vi "Example_Labview.vi"() -> ()   [LabVIEW 2019]
uses:
  <vilib>/myRIO/Common/Instrument Driver Framework/Utilities/typedefs/Analog Scaling Constants.ctl
  <vilib>/myRIO/Common/Instrument Driver Framework/Utilities/typedefs/Analog Scaling Constants List.ctl
  <vilib>/myRIO/Common/Instrument Driver Framework/myRIO v1.0/AO/typedefs/AO Channels Enum.ctl
  <vilib>/myRIO/Common/Instrument Driver Framework/myRIO v1.0/AO/typedefs/AO Channels List.ctl
  <vilib>/myRIO/Common/Instrument Driver Framework/Utilities/typedefs/Generic FPGA Reference.ctl
  <vilib>/myRIO/Common/Instrument Driver Framework/Utilities/typedefs/myRIO v1.0 Reference.ctl
  <vilib>/myRIO/Common/Instrument Driver Framework/Utilities/typedefs/Hardware Version Enum.ctl
  <vilib>/myRIO/Common/Instrument Driver Framework/Utilities/typedefs/myRIO Generic Hardware Reference.ctl
  <vilib>/myRIO/Instrument Drivers/Onboard IO/AO/typedefs/AO Reference.ctl
  <vilib>/userdefined/High Color/nirio_resource_hc.ctl
  <vilib>/myRIO/Common/Instrument Driver Framework/myRIO v1.0/AO/vis/myRIO v1.1 Open AO.vi
  <vilib>/myRIO/Instrument Drivers/Onboard IO/AO/vis/myRIO AO Open.xnode
  <vilib>/myRIO/Common/Instrument Driver Framework/myRIO v1.0/Encoder/typedefs/Encoder Signal Mode.ctl
  <vilib>/myRIO/Common/Instrument Driver Framework/myRIO v1.0/AI/typedefs/AI Channels Enum.ctl
  <vilib>/myRIO/Common/Instrument Driver Framework/myRIO v1.0/AI/typedefs/AI Channels List.ctl
  <vilib>/myRIO/Instrument Drivers/Onboard IO/AI/typedefs/AI Reference.ctl
  <vilib>/myRIO/Common/Instrument Driver Framework/myRIO v1.0/AI/vis/myRIO v1.1 Open AI.vi
  <vilib>/myRIO/Instrument Drivers/Onboard IO/AI/vis/myRIO AI Open.xnode
  <vilib>/Platform/TimedLoop/XDataNode/XDataNode.xnode
  <vilib>/Platform/TimedLoop/XDataNode/nitl_modes.ctl
  <vilib>/Platform/TimedLoop/XDataNode/XDNodeRunTimeDep.lvlib
  <vilib>/Platform/TimedLoop/XDataNode/wakeup.ctl
  <vilib>/Platform/TimedLoop/XDataNode/timing_clust.ctl
  <vilib>/Analysis/3filter.llb/Filter Passband Type.ctl
  <vilib>/Analysis/NI_AALBase.lvlib
  <vilib>/ptbypt/NI_PtbyPt.lvlib
  Shared VIs/TypeDef_TDMS_States.ctl
panel:
  out "Current [A]":dbl
  out "Voltage":dbl
  out "Time (ms)":dbl
  out "Velocity encoder LP [deg/s]":dbl
  out "Velocity unfiltered [deg/s]":dbl
  out "Force unfiltered [N]":dbl
  in  "File name":string
  in  "Stop saving data":bool
  in  "Save data?":bool
  out "Force [N]":dbl
  out "Force Chart":dbl(graph)
  out "Velocity [deg/s]":dbl
  out "Velocity Chart":dbl(graph)
  out "Position [deg]":dbl
  out "Position Chart":dbl(graph)
  in  "stop":bool
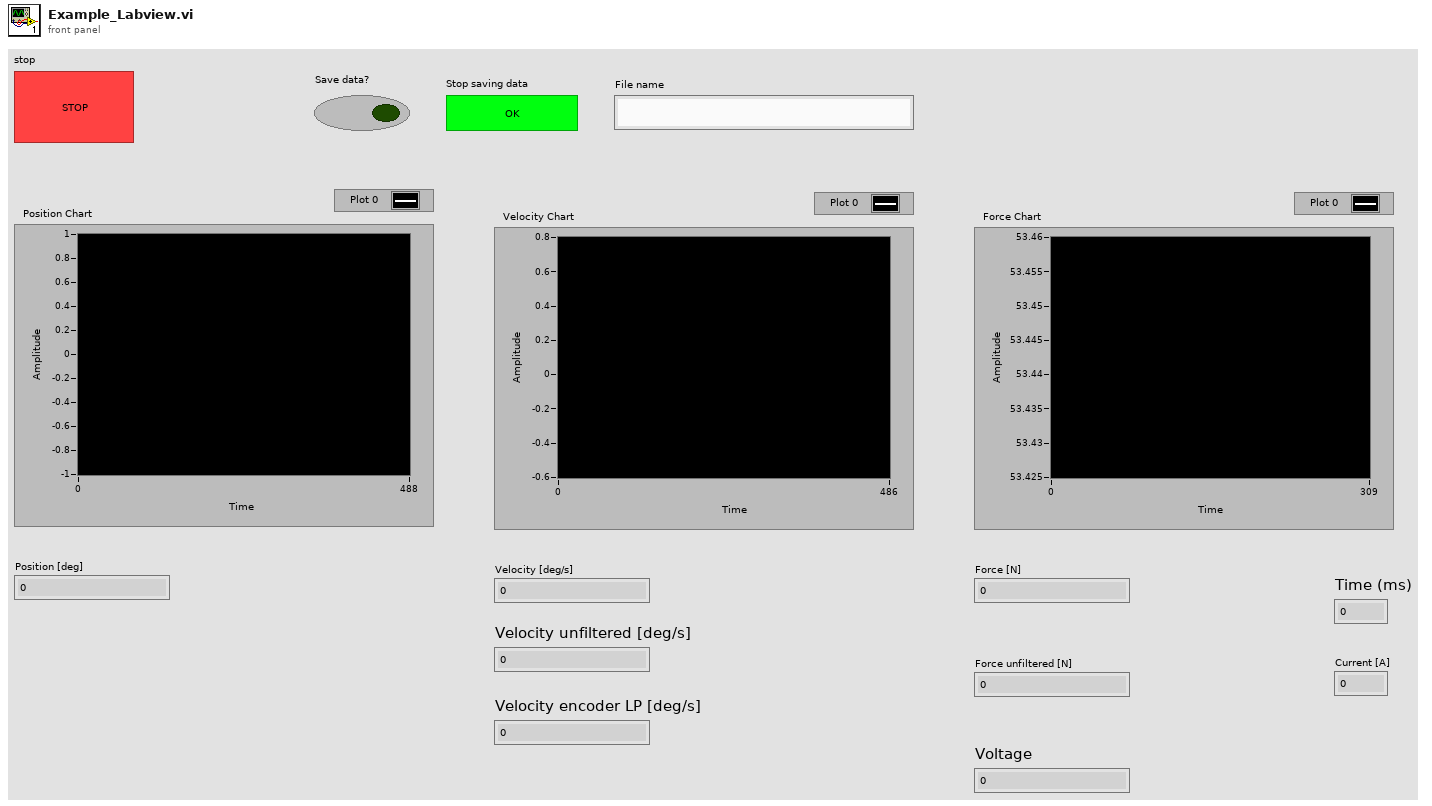
[diagram p1: front panel]
types:
  T1 = typedef "nirio_resource_hc.ctl" = tag
  T2 = typedef "Hardware Version Enum.ctl" = enum16{"Unknown", "myRIO-1900", "myRIO-1950", "roboRIO"}
  T3 = typedef "TypeDef_TDMS_States.ctl" = enum16{"Do Nothing", "Create", "Write", "Close"}
  T4 = enum16{"open", "open or create", "create or replace", "create", "open (read-only)"}
  T5 = typedef "XDNodeRunTimeDep.lvlib/timing_clust.ctl" = cluster{"Expected End [f-1]":u64, "Actual End [f-1]":u64, "Finished Late? [f-1]":bool, "Expected End [i-1]":u64, "Actual End [i-1]":u64, "Finished Late? [i-1]":bool, "Expected Start [i]":u64, "Actual Start [i]":u64, "Expected Start [f]":u64, "Actual Start [f]":u64, "Source Name":string, "Structure Name":string, "Period":i64, "Deadline":i64, "Offset":i64, "Start":i64, "Priority":i32, "Timeout":i32, "Mode":T6, "Wakeup Reason":T7, "Error":errorcluster, "Source Type":string, "Secondary Source Type":string, "Global End Time":u64, "Global Start Time":u64, "Frame Duration":u64, "Iteration Duration":u64, "Assigned CPU":i32, "I/O Scan Engine Mode":u32}
  T6 = typedef "XDNodeRunTimeDep.lvlib/nitl_modes.ctl" = enum32{"No Change", "Process missed periods, maintain original phase", "Discard missed periods, maintain original phase", "Process missed periods, ignore original phase", "Discard missed periods, ignore original phase"}
  T7 = typedef "XDNodeRunTimeDep.lvlib/wakeup.ctl" = enum32{"Normal", "Aborted", "Asynchronous wakeup", "Timing source error", "Timed loop error", "Timeout"}
  T8 = typedef "NI_AALBase.lvlib/Filter Passband Type.ctl" = enum32{"Lowpass", "Highpass", "Bandpass", "Bandstop"}
  T9 = typedef "Encoder Signal Mode.ctl" = enum16{"Quadrature phase signal", "Step and direction signal"}
  T10 = typedef "AO.lvlib/AO Reference.ctl" = cluster{"myRIO Reference":T11, "AO Channel List":T14, "AO Scaling Constant List":T16}
  T11 = typedef "myRIO Generic Hardware Reference.ctl" = cluster{"myRIO Model":T2, "myRIO Hardware Reference":T12}
  T12 = typedef "myRIO v1.0 Reference.ctl" = cluster{"Generic FPGA Reference":T13, "Allow multiple opens":bool}
  T13 = typedef "Generic FPGA Reference.ctl" = refnum<k20>
  T14 = typedef "AO Channels List.ctl" = T15[]
  T15 = typedef "AO Channels Enum.ctl" = enum16{"Not Connected", "AudioOut/Left", "AudioOut/Right", "C/AO0", "C/AO1", "A/AO0", "A/AO1", "B/AO0", "B/AO1"}
  T16 = typedef "Analog Scaling Constants List.ctl" = T17[]
  T17 = typedef "Analog Scaling Constants.ctl" = cluster{"LSB Weight (Volts)":dbl, "Offset (Volts)":dbl, "Signed?":bool}
  T18 = typedef "AI.lvlib/AI Reference.ctl" = cluster{"myRIO Reference":T11, "AI Channels List":T19, "AI Scaling Constants List":T16}
  T19 = typedef "AI Channels List.ctl" = T20[]
  T20 = typedef "AI Channels Enum.ctl" = enum16{"Not Connected", "AudioIn/Left", "AudioIn/Right", "C/AI0", "C/AI1", "A/AI0", "A/AI1", "A/AI2", "A/AI3", "B/AI0", "B/AI1", "B/AI2", "B/AI3", "AI/AI0", "AI/AI1", "AI/AI2", "AI/AI3"}
  T21 = typedef "Encoder.lvlib/Encoder Reference.ctl" = cluster{"myRIO Reference":T11, "Encoder Channels Enum":T22}
  T22 = typedef "Encoder Channels Enum.ctl" = enum16{"Not Connected", "C/ENC0", "C/ENC1", "A/ENC", "B/ENC", "DIO/ENC0", "DIO/ENC1", "DIO/ENC2", "DIO/ENC3", "DIO/ENC4"}
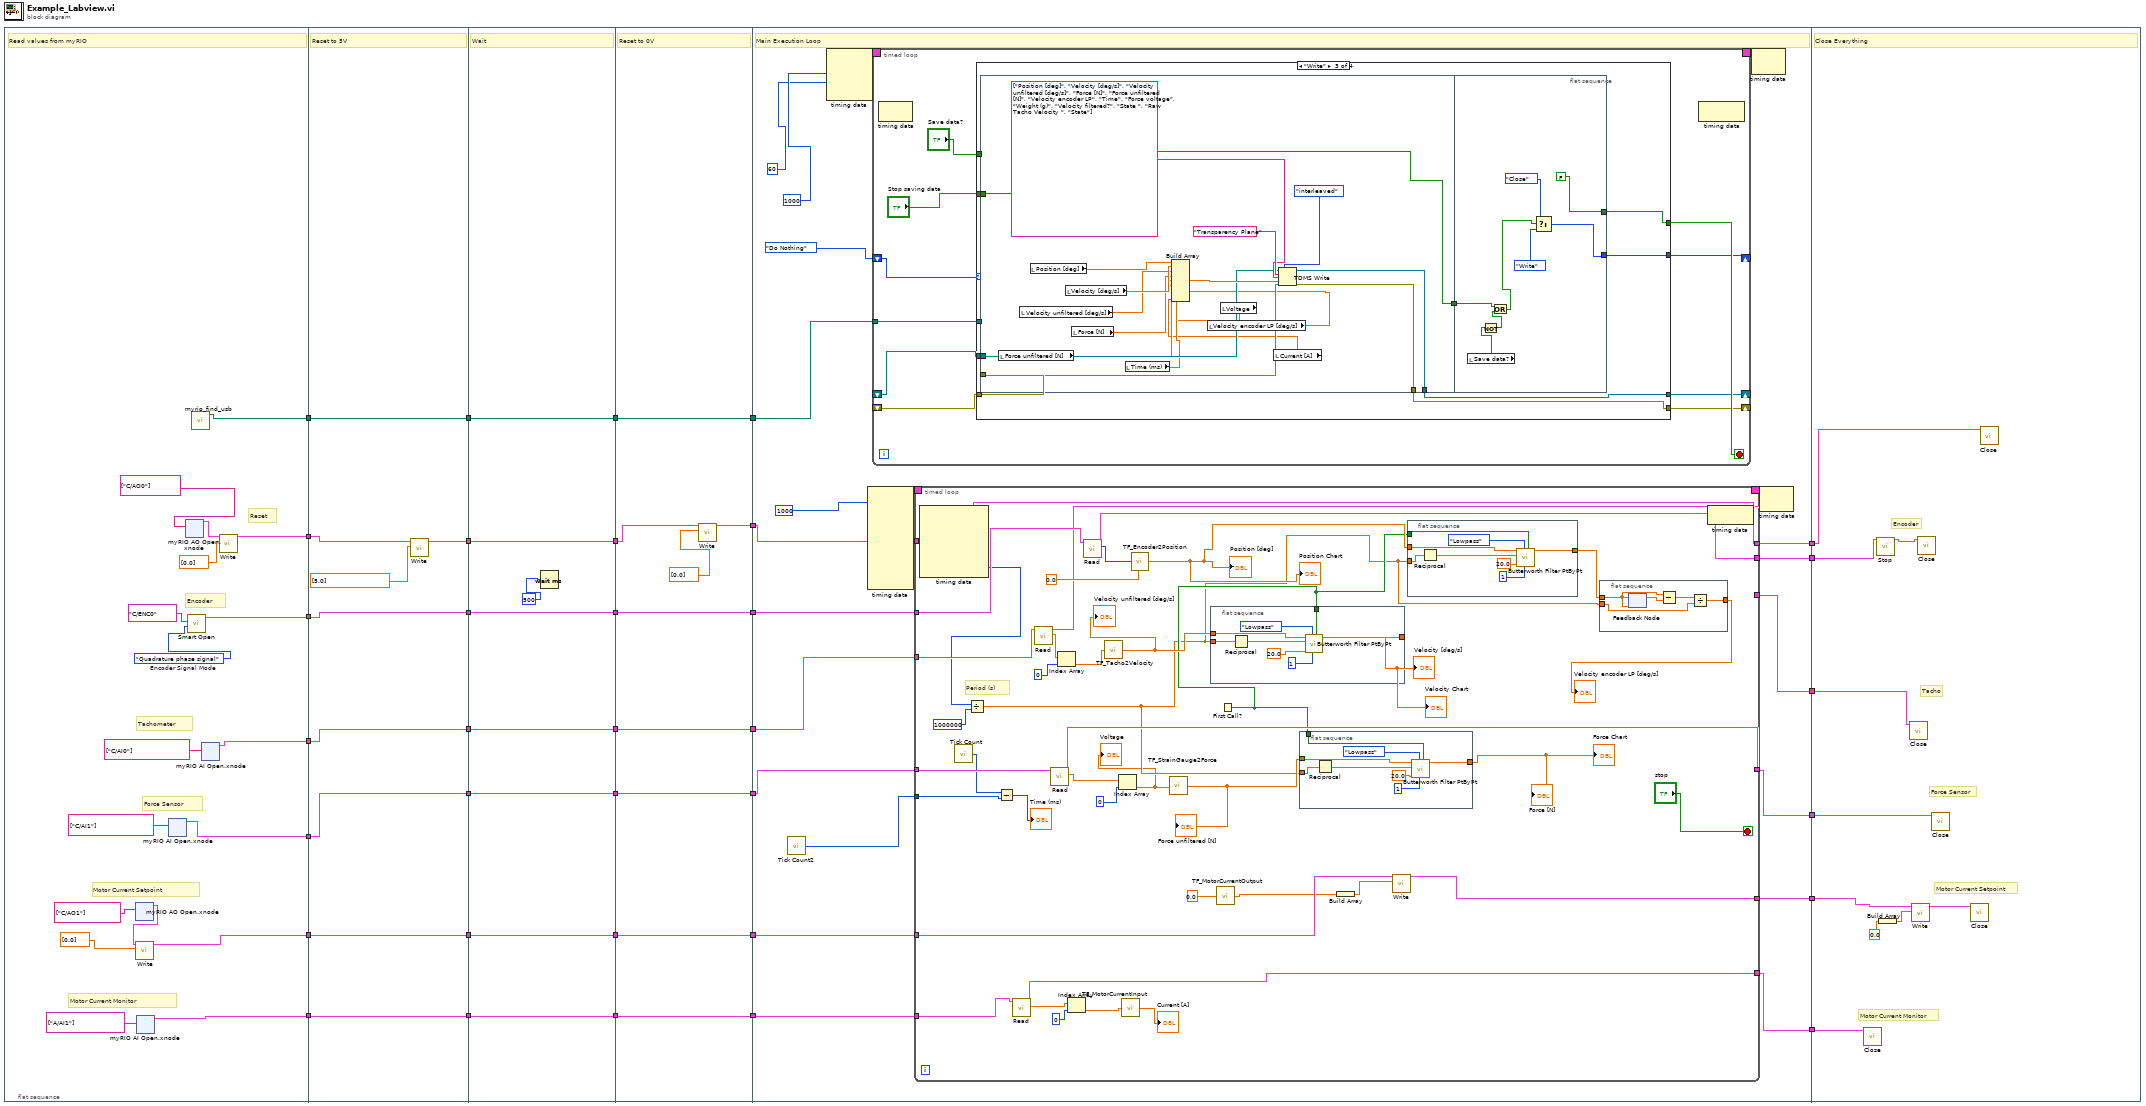
[diagram p0: block diagram]
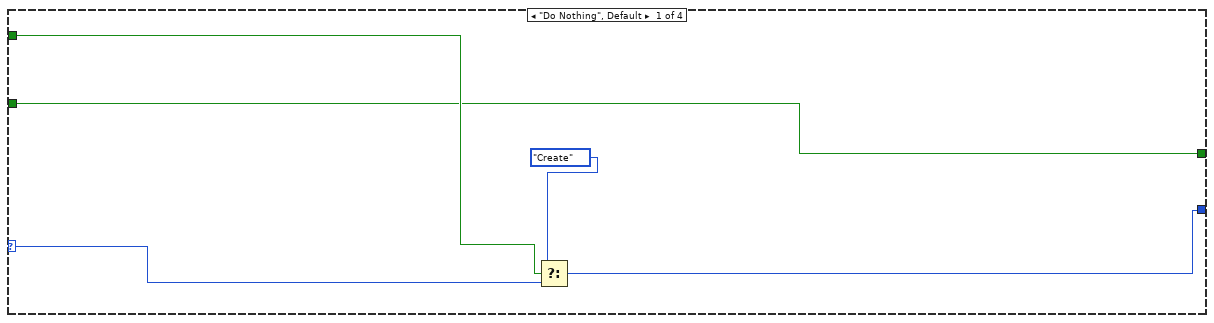
[diagram p2: hidden frame]
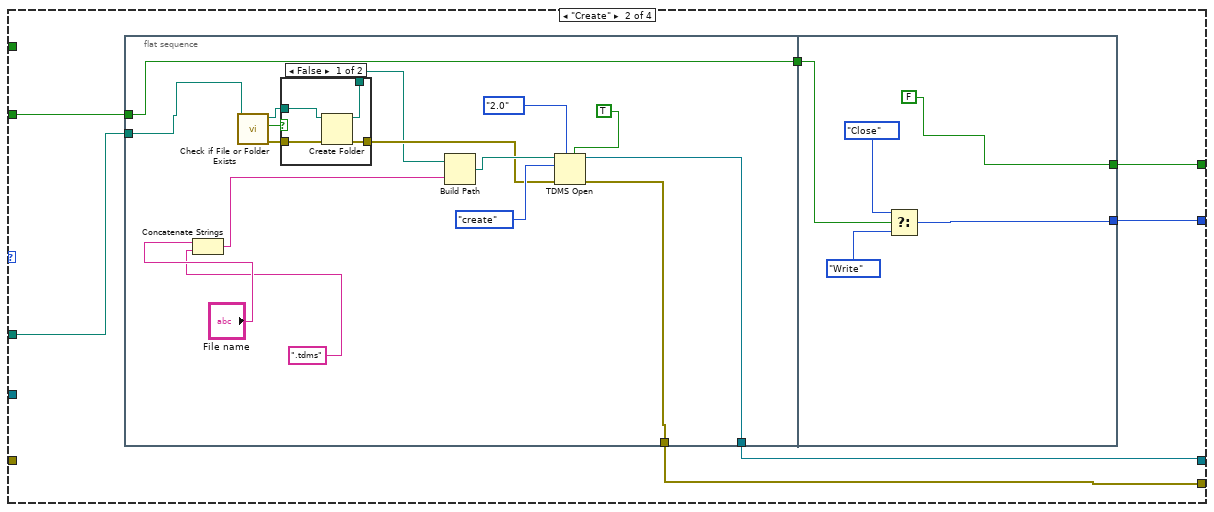
[diagram p3: hidden frame]
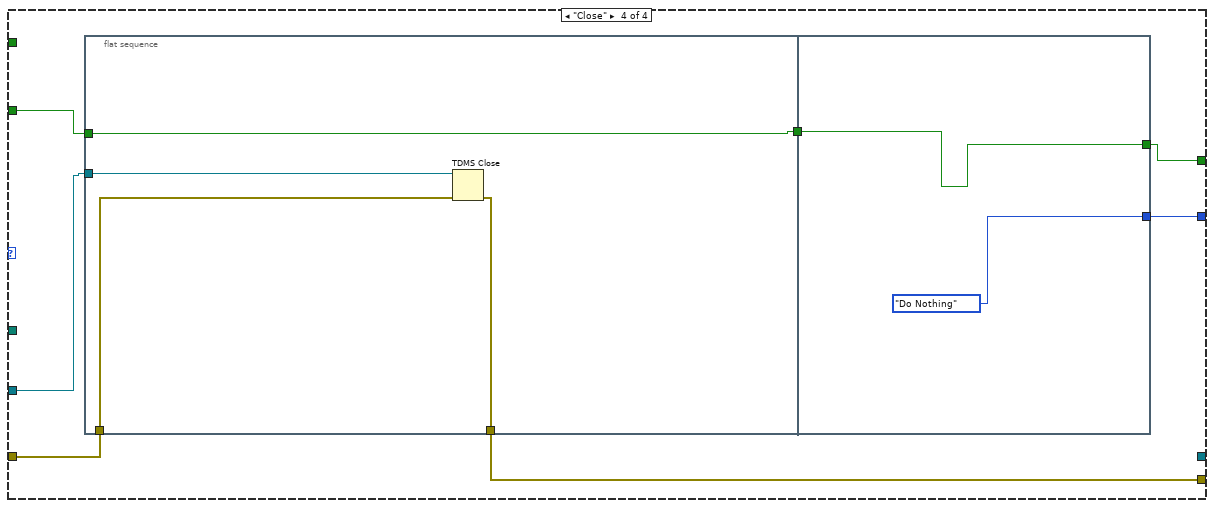
[diagram p5: hidden frame]
diagram:
  n1 = flat-sequence {
    tunnel: [w46] -> w34
    tunnel: [w45] -> w33
    tunnel: [w44] -> w32
    tunnel: [w43] -> w31
    tunnel: [w41] -> w21
    tunnel: [w37] -> w7
    tunnel: [w35] -> w2
    tunnel: w34 -> [w145]
    tunnel: w33 -> [w150]
    tunnel: w32 -> [w148]
    tunnel: w31 -> [w147]
    tunnel: [w149] -> w30
    tunnel: [w148] -> w25
    tunnel: [w147] -> w22
    tunnel: w21 -> [w146]
    tunnel: [w146] -> w18
    tunnel: [w145] -> w11
    tunnel: [w144] -> w8
    tunnel: w7 -> [w144]
    tunnel: [w143] -> w3
    tunnel: w2 -> [w143]
    tunnel: w30 -> [w158]
    tunnel: [w158] -> w29
    tunnel: [w157] -> w26
    tunnel: w25 -> [w157]
    tunnel: [w156] -> w23
    tunnel: w22 -> [w156]
    tunnel: [w155] -> w19
    tunnel: w18 -> [w155]
    tunnel: [w154] -> w12
    tunnel: w11 -> [w154]
    tunnel: [w153] -> w9
    tunnel: w8 -> [w153]
    tunnel: [w152] -> w4
    tunnel: w3 -> [w152]
    tunnel: w29 -> [w167]
    tunnel: [w166] -> w28
    tunnel: [w165] -> w27
    tunnel: w26 -> [w165]
    tunnel: [w164] -> w24
    tunnel: w23 -> [w164]
    tunnel: [w163] -> w20
    tunnel: w19 -> [w163]
    tunnel: [w162] -> w13
    tunnel: w12 -> [w162]
    tunnel: [w161] -> w10
    tunnel: w9 -> [w161]
    tunnel: [w160] -> w5
    tunnel: w4 -> [w160]
    tunnel: w28 -> [w187]
    tunnel: w27 -> [w185]
    tunnel: w24 -> [w183]
    tunnel: w20 -> [w182]
    tunnel: [w186] -> w17
    tunnel: [w184] -> w16
    tunnel: [w181] -> w15
    tunnel: [w180] -> w14
    tunnel: w13 -> [w177]
    tunnel: w10 -> [w172]
    tunnel: [w171] -> w6
    tunnel: w5 -> [w170]
    tunnel: [w169] -> w1
    tunnel: w17 -> [w380]
    tunnel: w16 -> [w378]
    tunnel: w15 -> [w377]
    tunnel: w14 -> [w376]
    tunnel: w6 -> [w372]
    tunnel: w1 -> [w371]
    frame #0 {
      w48 = Encoder_Signal_Mode."Quadrature phase signal"  # Encoder Signal Mode
      # "Motor Current Monitor"
      # "Motor Current Setpoint"
      # "Force Sensor"
      # "Tachometer"
      # "Encoder"
      # "Reset"
      # "Read values from myRIO"
      n2 = xnode "myRIO AO Open.xnode"("Channel Names"=tag[] ["C/AO1"]) -> ("AO Ref Out"=w39:T10)  [unwired: 2 in, 1 out]
      n3 = call <vilib>:"Write.vi"("Values"=dbl[] [0.0], "AO Ref In"=w39) -> ("AO Ref Out"=w37:T10)  [unwired: 7 in, 1 out]
      n4 = xnode "myRIO AI Open.xnode"("Channel Names"=tag[] ["A/AI1"]) -> ("AI Ref Out"=w35:T18)  [unwired: 2 in, 1 out]
      n5 = xnode "myRIO AI Open.xnode"("Channel Names"=tag[] ["C/AI1"]) -> ("AI Ref Out"=w41:T18)  [unwired: 2 in, 1 out]
      n6 = xnode "myRIO AO Open.xnode"("Channel Names"=tag[] ["C/AO0"]) -> ("AO Ref Out"=w51:T10)  [unwired: 2 in, 1 out]
      n7 = call <vilib>:"Smart Open.vi"("Encoder Signal Mode"=w48, "Channel Name"=tag "C/ENC0") -> ("Encoder Ref Out"=w44:T21)  [unwired: 8 in, 1 out]
      n8 = call "myrio_find_usb.vi"() -> ("Largest USB Partition Path"=w46:path)  [unwired: 9 in, 2 out]
      n9 = xnode "myRIO AI Open.xnode"("Channel Names"=tag[] ["C/AI0"]) -> ("AI Ref Out"=w43:T18)  [unwired: 2 in, 1 out]
      n10 = call <vilib>:"Write.vi"("Values"=dbl[] [0.0], "AO Ref In"=w51) -> ("AO Ref Out"=w45:T10)  [unwired: 7 in, 1 out]
    }
    frame #1 {
      # "Reset to 5V"
      n11 = call <vilib>:"Write.vi"("Values"=dbl[] [5.0], "AO Ref In"=w150) -> ("AO Ref Out"=w149:T10)  [unwired: 7 in, 1 out]
    }
    frame #2 {
      # "Wait"
      n12 = Wait (ms)(milliseconds to wait=500) -> ()  [unwired: 1 out]
    }
    frame #3 {
      # "Reset to 0V"
      n13 = call <vilib>:"Write.vi"("Values"=dbl[] [0.0], "AO Ref In"=w167) -> ("AO Ref Out"=w166:T10)  [unwired: 7 in, 1 out]
    }
    frame #4 {
      # "Main Execution Loop"
      n14 = call "Tick Count2"() -> ("Tick Count(mSec)"=w173:u32)
      n15 = node-c288(i64 1000 ("Period"), 60) -> (w179:T5)  [unwired: 2 in]
      n16 = node-c288(i64 1000 ("Period")) -> (w190:T5)  [unwired: 9 in]
      n17 = timed-loop {
        timing: w179 -> [_]
        timing-out: [_] -> w178
        shift-right: [w197] -> _
        shift-left: _ -> [w195]
        shift-right: [w196] -> _
        shift-left: _ -> [w194]
        tunnel: w177 -> [w193]
        shift-right: [w192] -> _
        shift-left: TypeDef_TDMS_States."Do Nothing" ("TDMS States") -> [w191]
        stop <- w199 stop-if-true
        n18 = node-c288() -> ()  [unwired: 1 in, 1 out]
        n19 = case shown="\"Write\"" w191 {
          selector: w191 -> [w203 _ _ _]
          tunnel: "Save data?" -> [w204 _ _ _]
          tunnel: [w202 w209 w241 w275] -> w199
          tunnel: "Stop saving data" -> [w202 w207 w242 w277]
          tunnel: [_ w212 w246 w276] -> w196
          tunnel: [_ w211 w245 _] -> w197
          tunnel: w195 -> [_ _ w244 w278]
          tunnel: w194 -> [_ _ w247 w279]
          tunnel: w193 -> [_ w210 _ _]
          tunnel: [w201 w206 w240 w274] -> w192
          frame "Do Nothing", Default {
            n20 = Select(t=TypeDef_TDMS_States."Create" ("TDMS States"), s=w204, f=w203) -> (s? t:f=w201:T3)
          }
          frame "Create" {
            n21 = flat-sequence {
              tunnel: [w217] -> w212
              tunnel: [w216] -> w211
              tunnel: w210 -> [w215]
              tunnel: [w213] -> w208
              tunnel: w207 -> [w213]
              tunnel: [FALSE ("Button :: Stop")] -> w209
              tunnel: w208 -> [w236]
              tunnel: [w235] -> w206
              frame #0 {
                n22 = Concatenate Strings("File name", ".tdms") -> (w225:string)
                n23 = call <vilib>:"Check if File or Folder Exists.vi"("path"=w215) -> ("error out"=w226:errorcluster, "file or folder exists?"=w228:bool, "dup path"=w227:path)  [unwired: 8 in]
                n24 = case shown="False" w228 {
                  tunnel: w227 -> [w232 w233]
                  tunnel: [w231 w234] -> w220
                  tunnel: w226 -> [w230 w234]
                  tunnel: [w229 w233] -> w214
                  frame False {
                    n25 = Create Folder(path (use dialog)=w232, error in=w230) -> (created path=w229:path, error out=w231:errorcluster)  [unwired: 1 in, 1 out]
                  }
                  frame True {
                  }
                }
                n26 = Build Path(base path=w214, name or relative path=w225) -> (appended path=w224:path)
                n27 = TDMS Open(5:TRUE, 7:enum16{"1.0", "2.0"}."2.0" ("file format version (2.0)"), 8:w220, 10:T4."create" ("operation (0:open)"), 11:w224) -> (0:w217:errorcluster, 3:w216:refnum<k34>)  [unwired: 2 in]
              }
              frame #1 {
                n28 = Select(t=TypeDef_TDMS_States."Close" ("TDMS States"), s=w236, f=TypeDef_TDMS_States."Write" ("TDMS States")) -> (s? t:f=w235:T3)
              }
            }
          }
          frame "Write" {
            n29 = flat-sequence {
              tunnel: w247 -> [w262]
              tunnel: [w258] -> w246
              tunnel: [w257] -> w245
              tunnel: w244 -> [w256]
              tunnel: [w255] -> w243
              tunnel: w242 -> [w255]
              tunnel: w243 -> [w271]
              tunnel: [FALSE ("Button :: Stop")] -> w241
              tunnel: [w266] -> w240
              frame #0 {
                n30 = local read "Force unfiltered [N]"() -> (w252:dbl)
                n31 = local read "Velocity unfiltered [deg/s]"() -> (w254:dbl)
                n32 = local read "Position [deg]"() -> (w265:dbl)
                n33 = local read "Velocity [deg/s]"() -> (w264:dbl)
                n34 = local read "Force [N]"() -> (w253:dbl)
                n35 = local read "Time (ms)"() -> (w250:dbl)
                n36 = local read "Velocity encoder LP [deg/s]"() -> (w251:dbl)
                n37 = local read "Voltage"() -> (w249:dbl)
                n38 = local read "Current [A]"() -> (w248:dbl)
                n39 = Build Array(w265, w264, w254, w253, w252, w251, w250, w249, w248) -> (w259:dbl[])
                n40 = TDMS Write(0:w256, 1:enum16{"decimated", "interleaved"}."interleaved" ("data layout (0:decimated)"), 5:"Transparency Plane" ("group name in (Untitled)"), 7:string[] ["Position [deg]", "Velocity [deg/s]", "Velocity unfiltered [deg/s]", "Force [N]", "Force unfiltered [N]", "Velocity encoder LP", "Time", "Force voltage", "Weight (g)", "Velocity filtered?", "State ", "Raw Tacho Velocity ", "State"], 9:w259, 11:w262) -> (4:w257:refnum<k34>, 15:w258:errorcluster)  [unwired: 2 out]
              }
              frame #1 {
                n41 = local read "Save data?"() -> (w272:bool)
                n42 = Not(x=w272) -> (.not. x?=w273:bool)
                n43 = Or(x=w271, y=w273) -> (x .or. y?=w268:bool)
                n44 = Select(t=TypeDef_TDMS_States."Close" ("TDMS States"), s=w268, f=TypeDef_TDMS_States."Write" ("TDMS States")) -> (s? t:f=w266:T3)
              }
            }
          }
          frame "Close" {
            n45 = flat-sequence {
              tunnel: w278 -> [w284]
              tunnel: [w283] -> w276
              tunnel: [w282] -> w280
              tunnel: w277 -> [w282]
              tunnel: w279 -> [w281]
              tunnel: [w285] -> w275
              tunnel: [TypeDef_TDMS_States."Do Nothing" ("TDMS States")] -> w274
              tunnel: w280 -> [w285]
              frame #0 {
                n46 = TDMS Close(8:w281, 11:w284) -> (0:w283:errorcluster)  [unwired: 1 out]
              }
              frame #1 {
              }
            }
          }
        }
        n47 = node-c288() -> ()  [unwired: 1 in, 1 out]
      }
      n48 = timed-loop {
        timing: w190 -> [_]
        timing-out: [_] -> w189
        tunnel: [w332] -> w186
        tunnel: w187 -> [w332]
        tunnel: w185 -> [w330]
        tunnel: [w329] -> w184
        tunnel: w183 -> [w327]
        tunnel: [w326] -> w180
        tunnel: w182 -> [w309]
        tunnel: [w319] -> w181
        tunnel: w173 -> [w306]
        tunnel: w172 -> [w302]
        tunnel: [w300] -> w171
        tunnel: w170 -> [w296]
        tunnel: [w295] -> w169
        stop <- "stop" stop-if-true
        # "Period (s)"
        n49 = node-c288() -> (w322:i64)  [unwired: 1 in, 6 out]
        n50 = call "Tick Count"() -> ("Tick Count(mSec)"=w307:u32)
        n51 = Divide(x=w322, y=1000000) -> (x/y=w312:dbl)
        n52 = Subtract(x=w307, y=w306) -> (x-y=→"Time (ms)":u32)
        n53 = call <vilib>:"Read.vi"("AI Ref In"=w296) -> ("Values"=w298:dbl[], "AI Ref Out"=w295:T18)  [unwired: 8 in, 1 out]
        n54 = call <vilib>:"Read.vi"("AI Ref In"=w327) -> ("Values"=w325:dbl[], "AI Ref Out"=w326:T18)  [unwired: 8 in, 1 out]
        n55 = call <vilib>:"Read.vi"("AI Ref In"=w309) -> ("Values"=w318:dbl[], "AI Ref Out"=w319:T18)  [unwired: 8 in, 1 out]
        n56 = Index Array(array=w325, index=0) -> (element=w328:dbl)
        n57 = Index Array(array=w298, index=0) -> (element=w297:dbl)
        n58 = call <vilib>:"Read.vi"("Encoder Ref In"=w330) -> ("Counter Value"=w334:i32, "Encoder Ref Out"=w329:T21)  [unwired: 6 in, 3 out]
        n59 = call "TF_Tacho2Velocity.vi"("Motor Velocity Tacho Value [V]"=w328) -> ("Motor Velocity Tacho [deg/s]"=w315:dbl)  [unwired: 4 in]
        "Velocity unfiltered [deg/s]" <- w315
        n60 = Index Array(array=w318, index=0) -> (element=w305:dbl)
        "Voltage" <- w305
        n61 = call "TF_MotorCurrentInput.vi"("Motor Current Monitor Value [V]"=w297) -> ("Current [A]"=→"Current [A]":dbl)
        n62 = call "TF_Encoder2Position.vi"("Counter Value"=w334, "Offset"=0.0) -> ("Position [deg]"=w314:dbl)  [unwired: 3 in]
        "Position Chart" <- w314
        "Position [deg]" <- w314
        n63 = call "TF_StrainGauge2Force.vi"("Strain Gauge Value [V]"=w305) -> ("Force [N]"=w316:dbl)  [unwired: 4 in]
        "Force unfiltered [N]" <- w316
        n64 = flat-sequence {
          tunnel: w315 -> [w363]
          tunnel: w312 -> [w361]
          tunnel: [w358] -> w321
          tunnel: w313 -> [w356]
          frame #0 {
            n65 = Reciprocal(x=w361) -> (1/x=w362:dbl)
            n66 = call <vilib>:"Butterworth Filter PtByPt.vi"("initialize"=w356, "order"=1, "filter type"=Filter_Passband_Type."Lowpass", "low cutoff freq: fl"=20.0, "sampling freq: fs"=w362, "x"=w363) -> ("Filtered x"=w358:dbl)  [unwired: 3 in, 1 out]
          }
        }
        n67 = call "TF_MotorCurrentOutput.vi"("Motor Current Setpoint [A]"=0.0) -> ("Motor Current Setpoint [V]"=w301:dbl)
        n68 = First Call?() -> (First Call?: T/F=w313:bool)
        n69 = flat-sequence {
          tunnel: w316 -> [w355]
          tunnel: [w350] -> w317
          tunnel: w312 -> [w349]
          tunnel: w313 -> [w348]
          frame #0 {
            n70 = Reciprocal(x=w349) -> (1/x=w354:dbl)
            n71 = call <vilib>:"Butterworth Filter PtByPt.vi"("initialize"=w348, "order"=1, "filter type"=Filter_Passband_Type."Lowpass", "low cutoff freq: fl"=20.0, "sampling freq: fs"=w354, "x"=w355) -> ("Filtered x"=w350:dbl)  [unwired: 3 in, 1 out]
          }
        }
        n72 = Build Array(w301) -> (w303:dbl[])
        n73 = call <vilib>:"Write.vi"("Values"=w303, "AO Ref In"=w302) -> ("AO Ref Out"=w300:T10)  [unwired: 7 in, 1 out]
        n74 = flat-sequence {
          tunnel: w314 -> [w342]
          tunnel: w313 -> [w338]
          tunnel: [w336] -> w311
          tunnel: w312 -> [w335]
          frame #0 {
            n75 = Reciprocal(x=w335) -> (1/x=w341:dbl)
            n76 = call <vilib>:"Butterworth Filter PtByPt.vi"("initialize"=w338, "order"=1, "filter type"=Filter_Passband_Type."Lowpass", "low cutoff freq: fl"=20.0, "sampling freq: fs"=w341, "x"=w342) -> ("Filtered x"=w336:dbl)  [unwired: 3 in, 1 out]
          }
        }
        n77 = flat-sequence {
          tunnel: [w345] -> w310
          tunnel: w311 -> [w344]
          tunnel: w312 -> [w343]
          frame #0 {
            n78 = feedback #1(w344) -> (w347:dbl)
            n79 = feedback-in #1(w344) -> ()
            n80 = Subtract(x=w344, y=w347) -> (x-y=w346:dbl)
            n81 = Divide(x=w346, y=w343) -> (x/y=w345:dbl)
          }
        }
        n82 = node-c288() -> ()  [unwired: 1 in, 1 out]
        "Velocity Chart" <- w321
        "Velocity [deg/s]" <- w321
        "Force Chart" <- w317
        "Force [N]" <- w317
        "Velocity encoder LP [deg/s]" <- w310
      }
      n83 = node-c288(w178) -> ()  [unwired: 1 out]
      n84 = node-c288(w189) -> ()  [unwired: 1 out]
    }
    frame #5 {
      # "Motor Current Monitor"
      # "Motor Current Setpoint"
      # "Force Sensor"
      # "Tacho"
      # "Encoder"
      # "Close Everything"
      n85 = call <vilib>:"Close.vi"("AI Ref In"=w371) -> ()  [unwired: 10 in, 1 out]
      n86 = call <vilib>:"Stop.vi"("Encoder Ref In"=w378) -> ("Encoder Ref Out"=w379:T21)  [unwired: 9 in, 1 out]
      n87 = Build Array(0.0) -> (w373:dbl[])
      n88 = call <vilib>:"Close.vi"("AI Ref In"=w376) -> ()  [unwired: 10 in, 1 out]
      n89 = call <vilib>:"Write.vi"("Values"=w373, "AO Ref In"=w372) -> ("AO Ref Out"=w375:T10)  [unwired: 7 in, 1 out]
      n90 = call <vilib>:"Close.vi"("Encoder Ref In"=w379) -> ()  [unwired: 10 in, 1 out]
      n91 = call <vilib>:"Close.vi"("AI Ref In"=w377) -> ()  [unwired: 10 in, 1 out]
      n92 = call <vilib>:"Close.vi"("AO Ref In"=w375) -> ()  [unwired: 10 in, 1 out]
      n93 = call <vilib>:"Close.vi"("AO Ref In"=w380) -> ()  [unwired: 10 in, 1 out]
    }
  }
